vi "getData.vi"() -> ()   [LabVIEW 2013]
uses:
  Global/measurementGlobal.vi
panel:
  out "Analogue Data (volts)":dbl[][](array[numeric])
  out "Error Status":bool
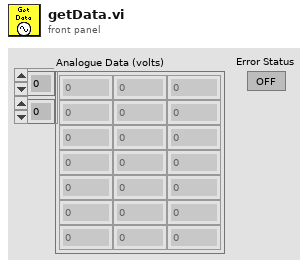
[diagram p1: front panel]
types:
  T1 = enum16{"New Measurement", "Post-process Raw Data"}
  T2 = cluster{dbl, dbl, "Input Sampling rate (Hz)":dbl}
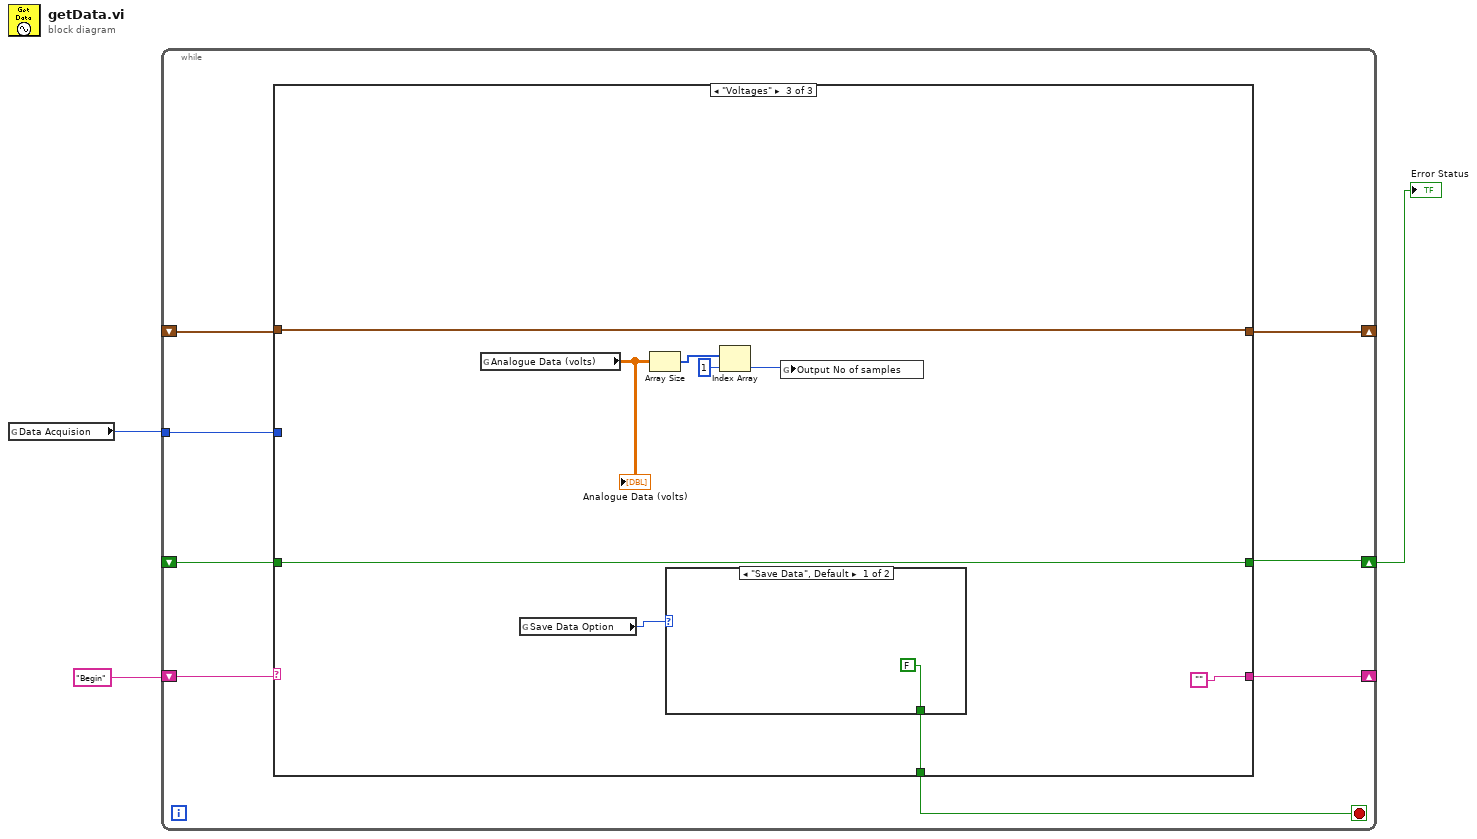
[diagram p0: block diagram]
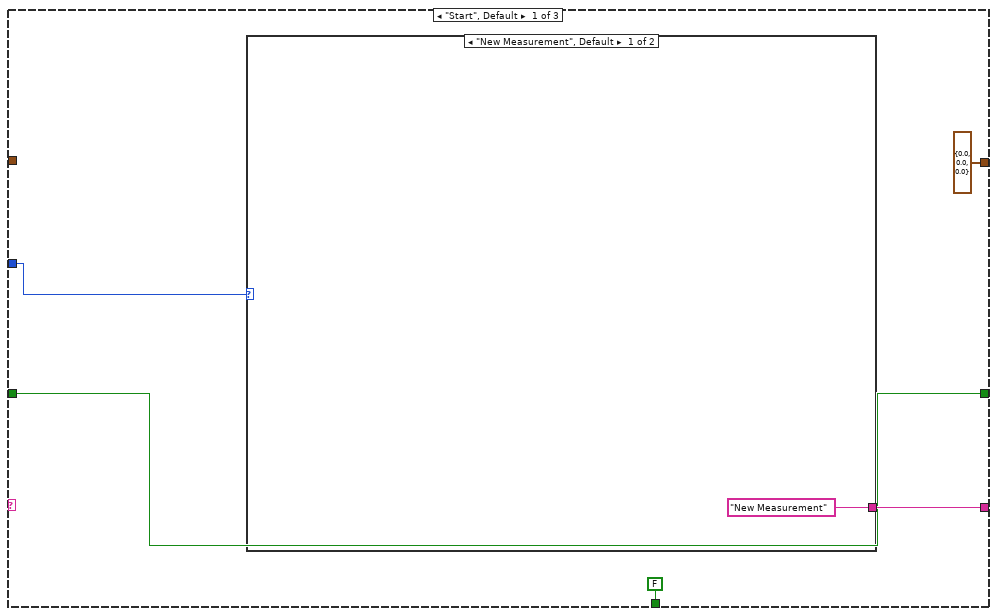
[diagram p2: hidden frame]
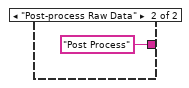
[diagram p3: hidden frame]
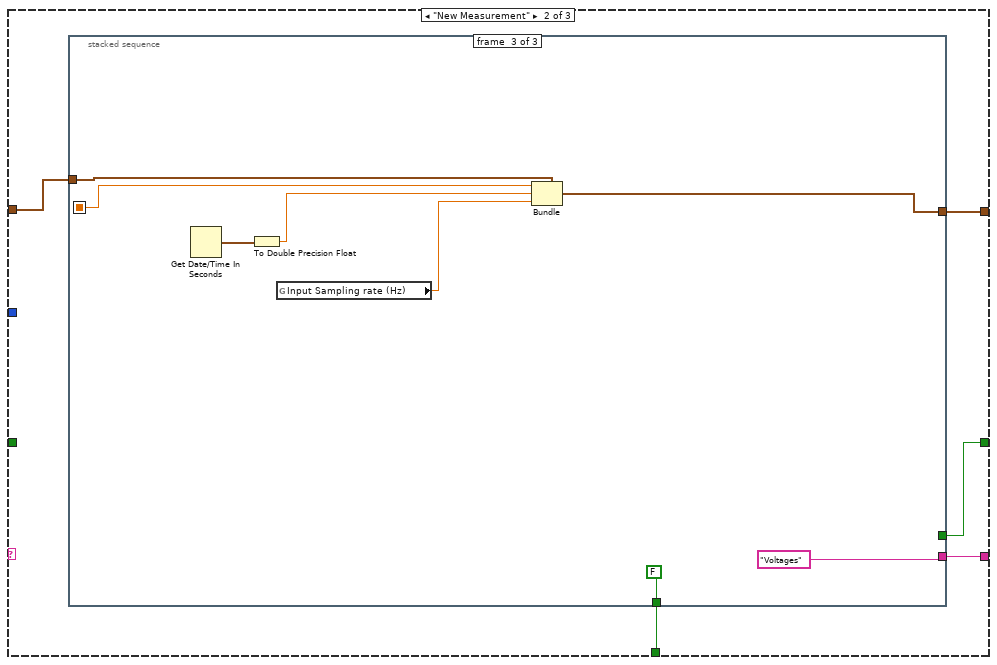
[diagram p4: hidden frame]
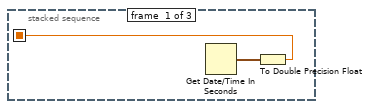
[diagram p5: hidden frame]
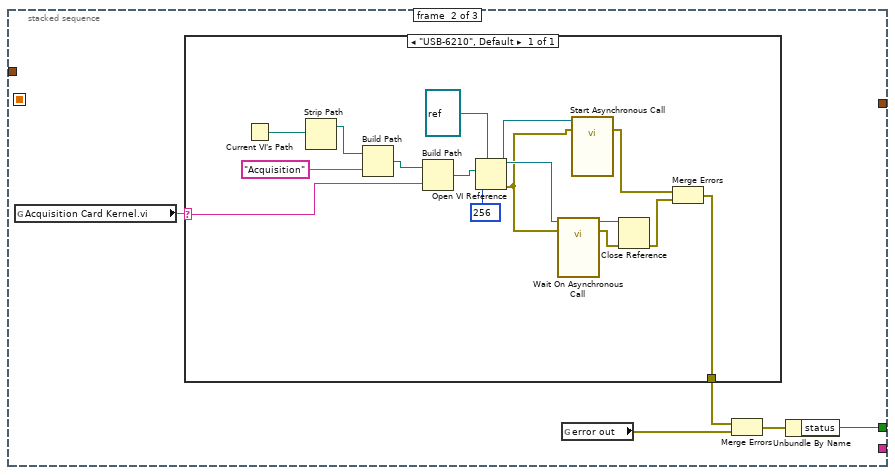
[diagram p6: hidden frame]
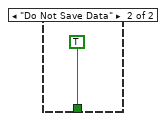
[diagram p7: hidden frame]
diagram:
  n1 = global read "measurementGlobal.vi" "Data Acquision"() -> (w2:T1)
  n2 = while {
    tunnel: w2 -> [w10]
    shift-right: [w4] -> _
    shift-left: "Begin" -> [w11]
    shift-right: [w9] -> w1
    shift-left: _ -> [w5]
    shift-right: [w8] -> _
    shift-left: _ -> [w7]
    stop <- w6 stop-if-true
    n3 = case shown="\"Voltages\"" w11 {
      tunnel: w10 -> [w15 _ _]
      tunnel: [w14 w20 ""] -> w4
      tunnel: [w13 w23 w55] -> w9
      tunnel: [T2 {0.0, 0.0, "Input Sampling rate (Hz)"=0.0} w22 w56] -> w8
      tunnel: w7 -> [_ w21 w56]
      tunnel: [FALSE w19 w57] -> w6
      tunnel: w5 -> [w13 _ w55]
      frame "Start", Default {
        n4 = case shown="\"New Measurement\", Default" w15 {
          tunnel: ["New Measurement" "Post Process"] -> w14
          frame "New Measurement", Default {
          }
          frame "Post-process Raw Data" {
          }
        }
      }
      frame "New Measurement" {
        n5 = stacked-sequence {
          seq-local: [w24 _ _] -> [_ _ w52]
          tunnel: [_ w26 _] -> w23
          tunnel: [_ _ w49] -> w22
          tunnel: w21 -> [_ _ w48]
          tunnel: [_ _ "Voltages"] -> w20
          tunnel: [_ _ FALSE] -> w19
          frame #0 {
            n6 = Get Date/Time In Seconds() -> (seconds since 1Jan1904=w25:timestamp)
            n7 = To Double Precision Float(number=w25) -> (double precision float=w24:dbl)
          }
          frame #1 {
            n8 = global read "measurementGlobal.vi" "Acquisition Card Kernel.vi"() -> (w30:string)
            n9 = case shown="\"USB-6210\", Default" w30 {
              selector: w30 -> [w41]
              tunnel: [w37] -> w29
              frame "USB-6210", Default {
                n10 = Current VI's Path() -> (path=w45:path)
                n11 = Strip Path(path=w45) -> (stripped path=w44:path)  [unwired: 1 out]
                n12 = Build Path(base path=w44, name or relative path="Acquisition") -> (appended path=w42:path)
                n13 = Build Path(base path=w42, name or relative path=w41) -> (appended path=w31:path)
                n14 = Open VI Reference(type specifier VI Refnum (for type only)=refnum<vi> refnum, vi path=w31, options=256) -> (vi reference=w36:refnum<vi>, error out=w35:errorcluster)  [unwired: 3 in]
                n15 = call-by-ref "Wait On Asynchronous Call"(reference=w36, error in=w35) -> (reference out=w40:refnum<vi>, error out=w39:errorcluster)  [unwired: 1 in, 1 out]
                n16 = call-by-ref "Start Asynchronous Call"(reference=w36, error in=w35) -> (error out=w34:errorcluster)  [unwired: 1 in, 2 out]
                n17 = Close Reference(reference=w40, error in (no error)=w39) -> (error out=w38:errorcluster)
                n18 = Merge Errors(w34, w38) -> (w37:errorcluster)
              }
            }
            n19 = global read "measurementGlobal.vi" "error out"() -> (w28:errorcluster)
            n20 = Merge Errors(w29, w28) -> (w27:errorcluster)
            n21 = Unbundle By Name(w27) -> ("status"=w26:bool)
          }
          frame #2 {
            n22 = Get Date/Time In Seconds() -> (seconds since 1Jan1904=w53:timestamp)
            n23 = To Double Precision Float(number=w53) -> (double precision float=w51:dbl)
            n24 = global read "measurementGlobal.vi" "Input Sampling rate (Hz)"() -> (w50:dbl)
            n25 = Bundle(cluster=w48, w52, w51, "Input Sampling rate (Hz)"=w50) -> (w49:T2)
          }
        }
      }
      frame "Voltages" {
        n26 = global read "measurementGlobal.vi" "Analogue Data (volts)"() -> (w62:dbl[][])
        "Analogue Data (volts)" <- w62
        n27 = global read "measurementGlobal.vi" "Save Data Option"() -> (w58:enum16{"Save Data", "Do Not Save Data"})
        n28 = Array Size(array=w62) -> (size(s)=w61:i32[])
        n29 = case shown="\"Save Data\", Default" w58 {
          tunnel: [FALSE TRUE] -> w57
          frame "Save Data", Default {
          }
          frame "Do Not Save Data" {
          }
        }
        n30 = Index Array(array=w61, index=1) -> (element=w59:i32)
        n31 = global write "measurementGlobal.vi" "Output No of samples"(w59) -> ()
      }
    }
  }
  "Error Status" <- w1
